vi "ShowTestresult.vi"() -> (3 "Terminated":bool)   [LabVIEW 2014]
uses:
  g_ChipData.vi
  g_Stop.vi
  g_CipHolderConstants.vi
panel:
  in  "OK":bool
  in  "Testresults":bool[][](array[boolean]) caption="Occupied"
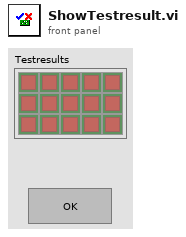
[diagram p1: front panel]
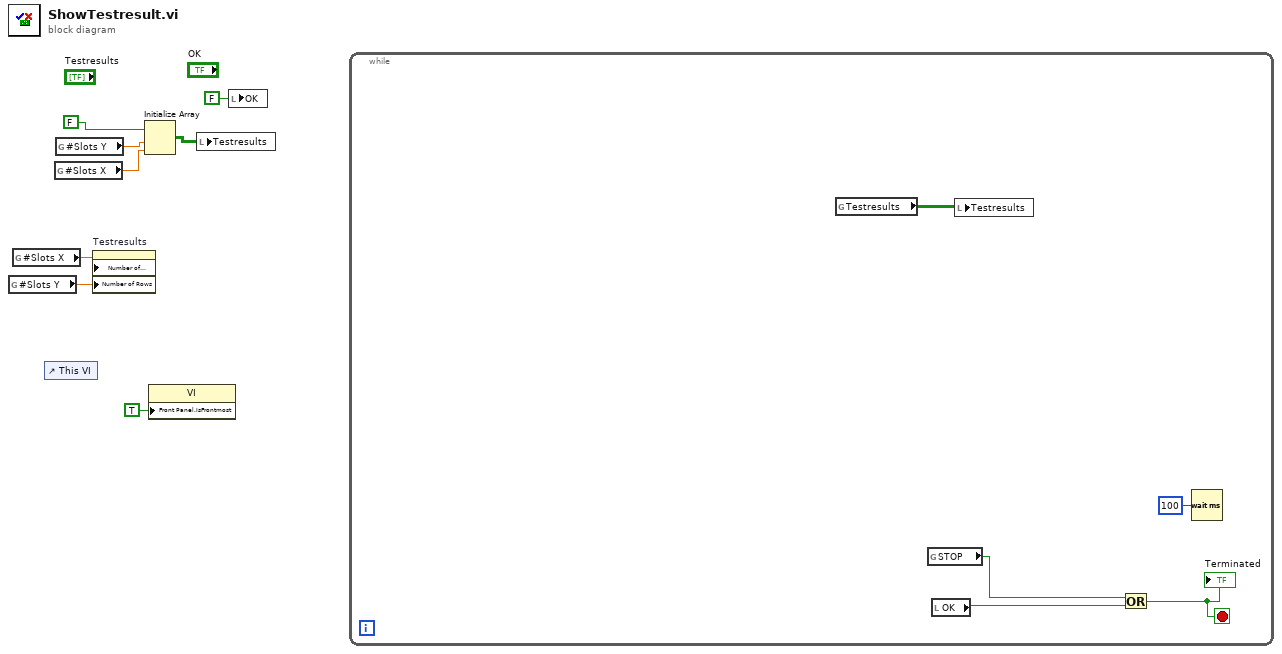
[diagram p0: block diagram]
diagram:
  n1 = global read "g_CipHolderConstants.vi" "#Slots Y"() -> (w4:dbl)
  n2 = global read "g_CipHolderConstants.vi" "#Slots X"() -> (w3:dbl)
  n3 = control-ref of="This VI"() -> ()  [unwired: 1 out]
  n4 = global read "g_CipHolderConstants.vi" "#Slots X"() -> (w7:dbl)
  n5 = global read "g_CipHolderConstants.vi" "#Slots Y"() -> (w8:dbl)
  n6 = property on="Testresults" class="Arr (strict)"("Number of Columns"=w3, "Number of Rows"=w4) -> ()  [unwired: 2 in, 2 out]
  n7 = Initialize Array(FALSE, w8, w7) -> (w5:bool[][])
  n8 = property class="VI"("Front Panel.IsFrontmost"=TRUE ("Front Panel Window:Is Frontmost")) -> ()  [unwired: 2 in, 2 out]
  n9 = local write "Testresults"(w5) -> ()
  n10 = local write "OK"(FALSE ("OK")) -> ()
  n11 = while {
    stop <- w11 stop-if-true
    n12 = global read "g_ChipData.vi" "Testresults"() -> (w13:bool[][])
    n13 = global read "g_Stop.vi" "STOP"() -> (w12:bool)
    n14 = local read "OK"() -> (w10:bool)
    n15 = local write "Testresults"(w13) -> ()
    n16 = Or(x=w12, y=w10) -> (x .or. y?=w11:bool)
    "Terminated" <- w11
    n17 = Wait (ms)(milliseconds to wait=u32 100) -> ()  [unwired: 1 out]
  }
